vi "for Kinematics.vi"(6 "constant":cluster{"d1":dbl, "a2":dbl, "a3":dbl}={"d1"=100.0, "a2"=67.0, "a3"=120.0}, 9 "theta3a":dbl, 10 "theta2a":dbl, 11 "theta1a":dbl) -> (1 "Pz":dbl, 2 "Py":dbl, 3 "Px":dbl)   [LabVIEW 2017]
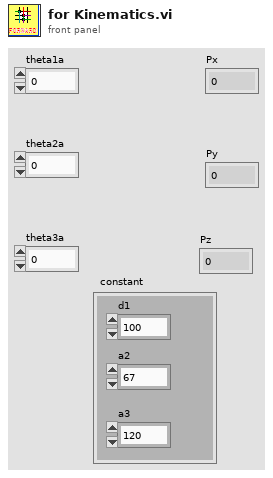
[diagram p1: front panel]
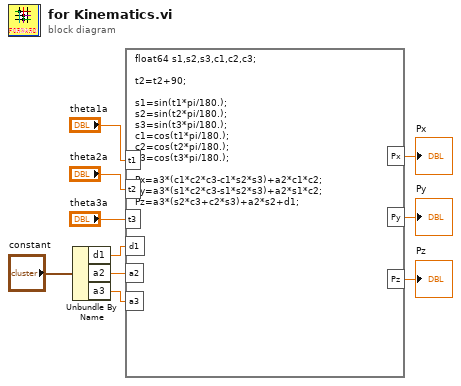
[diagram p0: block diagram]
diagram:
  n1 = Unbundle By Name("constant") -> ("d1"=w9:dbl, "a2"=w8:dbl, "a3"=w7:dbl)
  n2 = formula code="float64 s1,s2,s3,c1,c2,c3;\n\nt2=t2+90;\n\ns1=sin(t1*pi/180.);\ns2=sin(t2*pi/180.);\ns3=sin(t3*pi/180.);\nc1=cos(t1*pi/180.);\nc2=cos(t2*pi/180.);\nc3=cos(t3*pi/180.);\n\nPx=a3*(c1*c2*c3-c1*s2*s3)+a2*c1*c2;\nPy=a3*(s1*c2*c3-s1*s2*s3)+a2*s1*c2;\nPz=a3*(s2*c3+c2*s3)+a2*s2+d1;"("t1"="theta1a", "t2"="theta2a", "t3"="theta3a", "d1"=w9, "a2"=w8, "a3"=w7) -> ("Px"=→"Px":dbl, "Py"=→"Py":dbl, "Pz"=→"Pz":dbl)
